vi "CVT Enum GetDescription.vi"(8 "error in (no error)":errorcluster, 11 "Tag Name":string) -> (0 "error out":errorcluster, 2 "Tag Label":string)   [LabVIEW 2016]
uses:
  <vilib>/NI/Current Value Table/Compatibility/_SubVIs/TypeDefs/cvt_TagList Methods.ctl
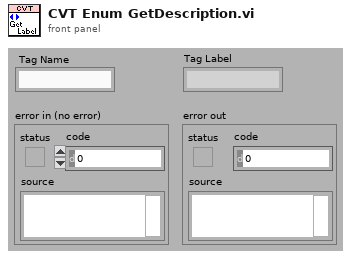
[diagram p1: front panel]
types:
  T1 = typedef "cvt_TagList Methods.ctl" = enum16{"init", "getindex", "getdesc", "getlist"}
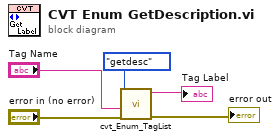
[diagram p0: block diagram]
diagram:
  n1 = call <vilib>:"cvt_Enum_TagList.vi"("error in (no error)"="error in (no error)", "Tag Name"="Tag Name", "Method"=cvt_TagList_Methods."getdesc") -> ("error out"=→"error out":errorcluster, "Tag Description"=→"Tag Label":string)  [unwired: 1 in, 6 out]
